vi "CONV String to 2D Integer.vi"(0 "String":string, 1 "Delimiters (,;)":string=",;") -> (6 "2-D Integer":i32[][](array[numeric]))   [LabVIEW 2012]
doc: "This routine converts a string list to a 2-D I32 Integer Array. There should be exactly 2 characters in the Delimiters field. The first is the Column delimiter, and the Second is the Row delimiter.\n\nExample:\n\nString: 1,2,3;4,5,6\nDelimiters: ,;\n\nOutput\n\n1 2 3\n4 5 6"
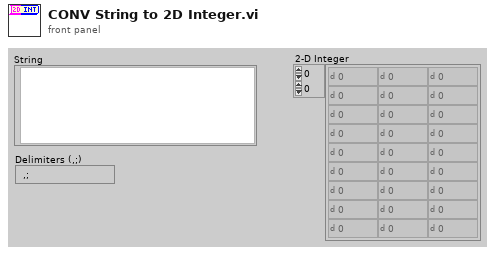
[diagram p1: front panel]
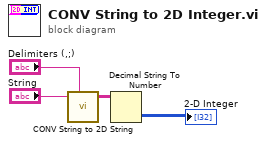
[diagram p0: block diagram]
diagram:
  n1 = call "CONV String to 2D String.vi"("String"="String", "Delimiters (,;)"="Delimiters (,;)") -> ("2-D String"=w2:string[][])  [unwired: 7 out]
  n2 = Decimal String To Number(string=w2) -> (number=→"2-D Integer":i32[][])  [unwired: 3 out]
